vi "PH_Beamline.set Switch State in GUI.vi"(0 "i ref in":refnum<vi>, 1 "Boolean GUI Ref":refnum<vi>, 2 "Picture GUI Ref":refnum<vi>, 3 "Status":T1 items=["no info", "off/false/out", "on/true/in", "Failure", "Alarm", "Status 1", "Status 2", "Status 3"], 4 "no Link?":bool, 5 "error in (no error)":errorcluster) -> (14 "i ref out":refnum<vi>, 19 "error out":errorcluster)   [LabVIEW 2014, in "PH_Beamline.lvlib"]
doc: "This VI writes the incoming information about switches to the GUI."
uses:
  PH_Beamline.lvlib
  PH_StatusHandler/PH_StatusHandler.Status.ctl
  PH_BL-Master/PH_BL-Master.Shutter State.ctl
  PH_Beamline.Switch Instances.ctl
  PH_Common/Picture/PH_Picture.Alignment.ctl
  PH_Common/PH_Common.lvlib
  PH_StatusHandler/PH_StatusHandler.lvlib
  PH_Switch/PH_Switch.lvlib
  PH_Beamline_Common/PH_Beamline_Common.lvlib
  PH_BL-Master/PH_BL-Master.lvlib
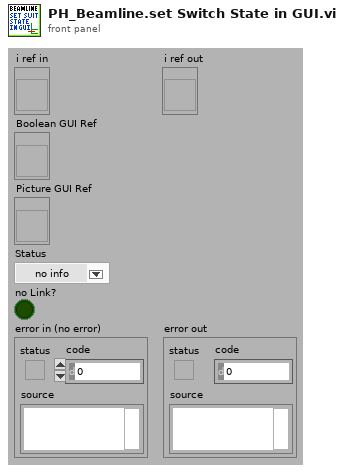
[diagram p1: front panel]
types:
  T1 = typedef "PH_StatusHandler.lvlib/PH_StatusHandler.Status.ctl" = i16
  T2 = typedef "PH_BL-Master.lvlib/PH_BL-Master.Shutter State.ctl" = enum16{"No Link", "No Info", "In", "Out", "in between"}
  T3 = typedef "PH_Beamline.lvlib/PH_Beamline.Switch Instances.ctl" = string
  T4 = typedef "PH_Common.lvlib/PH_Picture.Alignment.ctl" = enum16{"neutral", "left", "right", "up", "down", "vertical", "horizontal", "left down to right up", "left up to right down"}
  T5 = typedef "PH_Beamline.lvlib/PH_Beamline.i attribute.ctl" = cluster{"GUI Refs":cluster{"PA ok":refnum<vi>, "MA ok":refnum<vi>, "fs FE ok":refnum<vi>, "ns FE ok":refnum<vi>, "PA ED ok":refnum<vi>, "MAS ok":refnum<vi>, "Booster ok":refnum<vi>, "Mirrortower ok":refnum<vi>, "In.-Box ok":refnum<vi>, "Compressor ok":refnum<vi>, "Experiment LB ok":refnum<vi>, "Experiment LL ok":refnum<vi>, "PHELIX_Beckhoff_Watchdog":refnum<vi>, "Shutters closed":refnum<vi>, "uOPA ok":refnum<vi>, "Vacuum no shotcond Comp LB":refnum<vi>}, "Refs BL MA":refnum<vi>[], "Refs BL MA-IB":refnum<vi>[], "Refs BL fs":refnum<vi>[], "Refs BL PA ED":refnum<vi>[], "Refs BL MAS":refnum<vi>[], "Refs BL Boo":refnum<vi>[], "Refs BL ns":refnum<vi>[], "Refs BL Mirrortower":refnum<vi>[], "Refs BL Compressor":refnum<vi>[], "Refs BL Exp LB":refnum<vi>[], "Radiation Safety":cluster{"Exp Laserbay":cluster{"Ref Op Mode":refnum<vi>, "Ref Laserbay evacuated":refnum<vi>, "Tagname LB evacuated":string, "Shot Mode":T6, "Laserbay evacuated?":i32, "Tagname HV room locked":string, "HV room locked?":i32, "Ref HV room locked":refnum<vi>, "Tagname bridged?":string, "Ref Bridge":refnum<vi>, "I<1E18W/cm²":bool}, "Exp Laserlab":cluster{"Ref Op Mode":refnum<vi>, "Ref Laserlab evacuated":refnum<vi>, "Tagname LL evacuated":string, "Shot Mode":T6, "Laserlab evacuated?":i32, "Tagname bridged?":string, "Ref Bridge":refnum<vi>, "I<1E18W/cm²":bool}}, "Refs BL LL":refnum<vi>[], "PP Igni Heating GUI Refs":refnum<vi>[], "PP Igni Heating Tagnames ":string[], "Refs BL PA":cluster{"undelayed Line before Shutter":refnum<vi>[], "undelayed Line after Shutter":refnum<vi>[], "before Bypass":refnum<vi>[], "delayed Line before Shutter":refnum<vi>[], "delayed Line after Shutter":refnum<vi>[], "before Shutter Input":refnum<vi>[], "after Shutter Input":refnum<vi>[], "Bypass":refnum<vi>[], "before Shutter Exit":refnum<vi>[], "after Shutter Exit":refnum<vi>[], "to MA":refnum<vi>[], "to Lab":refnum<vi>[]}, "BL":cluster{"YLF_BL_Status":i32, "fs_BL_Status":i32, "fs_YLF_BL_Status":i32, "ns_BL_Status":i32, "PA_Input_BL_Status":i32, "PA_UnDelay_BL_Status":i32, "PA_Delay_BL_Status":i32, "PA_BL_Status":i32, "PA_Bypass_BL_Status":i32, "PA_Exit_BL_Status":i32, "PA_LL_BL_Status":i32, "LL_BL_Status":i32, "PA_MA_BL_Status":i32, "MA_Exit_BL_Status":i32, "MA_Z6_BL_Status":i32, "Z6_BL_Status":i32, "MA_LB_BL_Status":i32, "LB_TB2_BL_Status":i32, "PA_before_Bypass_BL_Status":i32, "LB_TB3_BL_Status":i32}, "State Subsystems":cluster{"PA":bool, "MA":bool, "ns FE":bool, "fs FE":bool, "PA ED":bool, "In.-Box":bool, "MAS":bool, "Booster":bool, "Mirrortower":bool, "Compressor":bool, "Experiment LB":bool, "Experiment LL":bool, "uOPA":bool}, "Status Subscriber Information":T7, "Refs BL uOPA":refnum<vi>[], "PA_Input_2_Beam_6PWpGUI not linked?":bool, "PA_Input_Delay_6PGUI not linked?":bool, "Settings":T10}
  T6 = typedef "PH_Beamline.lvlib/PH_Beamline.Operation Mode.ctl" = i32
  T7 = typedef "PH_Beamline.lvlib/PH_Beamline.Status Subscriber Information.ctl" = cluster{"fs Swich YLF":T8, "fs Exit Shutter":T8, "ns Exit Shutter":T8, "PA Input Shutter":T8, "PA PC WP":T8, "PA PC WP 2":T8, "PA Bypass In":T8, "PA Bypass Out":T8, "PA CH 1":T8, "PA delayed":T8, "PA non delayed":T8, "PA Exit Shutter":T8, "PA Switch Lab":T8, "PA Bridge CH Input MA":T8, "MA Diffusor IB":T8, "MA IB Ready":T8, "MA CH 1":T8, "MA CH 2":T8, "MA CH 3":T8, "MA CH 4":T8, "MA Shutter Align Cam":T8, "MA Position MM5":T8, "Calorimeter Switch":T8, "BL Z6 CH 9":T8, "BL Z6 Beamdump":T8, "BL Z6 Shutter":T8, "COS Sensitivity Switch":T8, "Exp LB Shutter":T8, "Exp LB TB 2":T8, "Exp LB TB 3":T8, "PA LL Input CH":T8, "PA LL Output CH":T8, "LL Comp Input Shutter":T8, "LL Comp Output Shutter":T8, "LL Comp FF Shutter":T8, "Exp LL Shutter":T8, "MA IM In IB":T8, "MA IM Out IB":T8, "MA DB In IB":T8, "MA DB Out IB":T8, "Exp LB Shutter Interlock":T8, "Exp LL Shutter Interlock":T8, "MM1 Force Sensor":T8}
  T8 = typedef "PH_BL-Master.lvlib/PH_BL-Master.Status Subscriber Information.ctl" = cluster{"Index of element":i32, "Attributeset":T9}
  T9 = typedef "PH_BL-Master.lvlib/PH_BL-Master.Attribute Set.ctl" = enum16{"Boolean Status Service Subscriber", "Picture Status Service Subscriber"}
  T10 = typedef "PH_Beamline_Chief.lvlib/PH_Beamline_Chief.Settings.ctl" = cluster{"PA Doublepass Mode":bool, "Compressor Vaccuum LB not relevant":bool, "Windowshutter TB2 not relevant":bool, "Windowshutter TB3 not relevant":bool}
  T11 = typedef "PH_BL-Master.lvlib/PH_BL-Master.i attribute.ctl" = cluster{"Remote controlled":bool, "Boolean Condition Service Subscriber":refnum<vi>[], "Picture Condition Service Subscriber":refnum<vi>[], "R2S":cluster{"GUI Ref":refnum<vi>, "State":bool}, "Vacua":cluster{"GUI Ref":refnum<vi>, "Limit":dbl, "Curr Value":dbl, "in range":bool}[], "O2 Inspection":cluster{"GUI Ref":refnum<vi>, "Concentration":dbl, "State":T1}[], "Boolean Status Service Subscriber":cluster{"GUI Ref":refnum<vi>, "Status":T1, "no Link?":bool, "Status Subscriber Class":T12}[], "Picture Status Service Subscriber":cluster{"GUI Ref":refnum<vi>, "Status":T1, "no Link?":bool, "Status Subscriber Class":T12}[], "6P 4Q Service Subscriber":cluster{"GUI Ref":refnum<vi>, "Selector":T13, "no Link?":bool}[], "Index of latest 6P 4Q changing Instance":i32, "Index of latest Picture Status changing Instance":i32, "Index of latest Boolean Status changing Instance":i32, "Vision ID on same Node":string, "Start Phase over?":bool, "GUI Ref Delete":refnum<vi>}
  T12 = typedef "PH_BL-Master.lvlib/PH_BL-Master.Status Subscriber Class.ctl" = enum16{"unknown", "Switch", "BB", "6P Switch", "Switch GUI", "Switch and 6P State", "Force Sensor"}
  T13 = typedef "PH_4_Pos_Selector.lvlib/PH_4_Pos_Selector.Position Selector.ctl" = u16
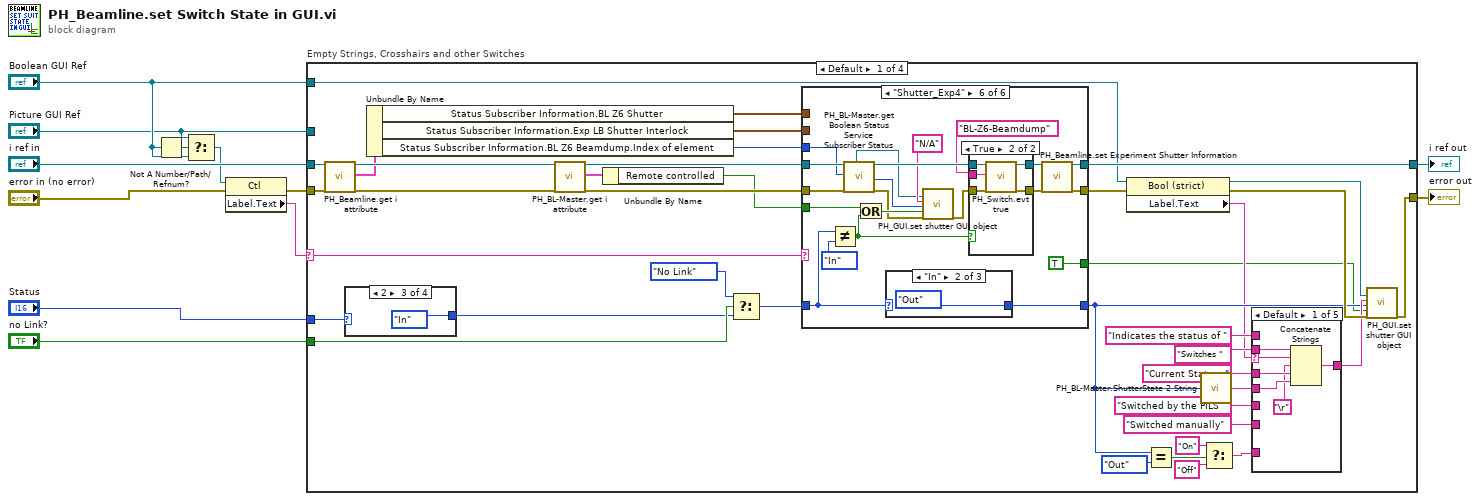
[diagram p0: block diagram]
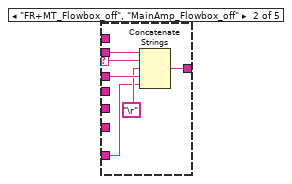
[diagram p2: hidden frame]
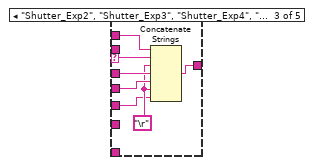
[diagram p3: hidden frame]
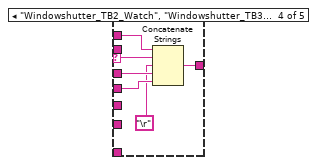
[diagram p4: hidden frame]
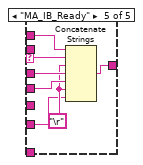
[diagram p5: hidden frame]
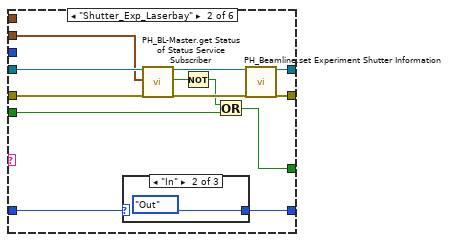
[diagram p7: hidden frame]
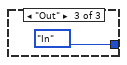
[diagram p9: hidden frame]
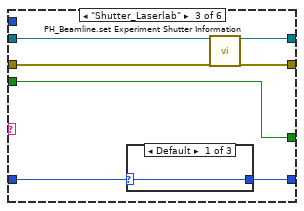
[diagram p10: hidden frame]
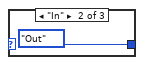
[diagram p11: hidden frame]
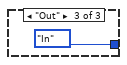
[diagram p12: hidden frame]
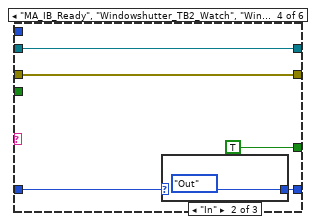
[diagram p13: hidden frame]
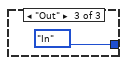
[diagram p15: hidden frame]
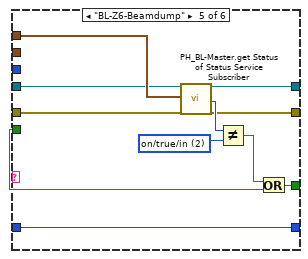
[diagram p16: hidden frame]
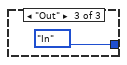
[diagram p18: hidden frame]
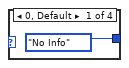
[diagram p20: hidden frame]
diagram:
  n1 = Not A Number/Path/Refnum?(number/path/refnum="Boolean GUI Ref") -> (NaN/Path/Refnum?=w4:bool)
  n2 = Select(t="Picture GUI Ref", s=w4, f="Boolean GUI Ref") -> (s? t:f=w3:refnum<vi>)
  n3 = property class="Ctl"(reference=w3, error in="error in (no error)") -> (error out=w1:errorcluster, "Label.Text"=w2:string)  [unwired: 1 out]
  n4 = case "Empty Strings, Crosshairs and other Switches" shown="Default" w2 {
    selector: w2 -> [w43 _ w178 w192]
    tunnel: w1 -> [w51 w168 w174 w185]
    tunnel: "i ref in" -> [w19 w172 w181 w193]
    tunnel: "Status" -> [w50 w171 w180 w190]
    tunnel: "no Link?" -> [w49 w170 _ _]
    tunnel: [w48 w173 w182 w194] -> w11
    tunnel: [w47 w172 w181 w193] -> w10
    tunnel: "Boolean GUI Ref" -> [w25 _ _ _]
    tunnel: "Picture GUI Ref" -> [_ w169 w175 w186]
    frame Default {
      n5 = call "PH_Beamline.get i attribute.vi"("i ref in"=w19, "error in (no error)"=w51) -> ("i ref out"=w18:refnum<vi>, "i attribute"=w17:T5, "error out"=w20:errorcluster)  [unwired: 15 in]
      n6 = case shown="2" w50 {
        tunnel: [PH_BL-Master.Shutter_State."No Info" ("Shutter State") PH_BL-Master.Shutter_State."Out" ("Shutter State") PH_BL-Master.Shutter_State."In" ("Shutter State") PH_BL-Master.Shutter_State."in between" ("Shutter State")] -> w45
        frame 0, Default {
        }
        frame 1 {
        }
        frame 2 {
        }
        frame 5 {
        }
      }
      n7 = Unbundle By Name(w17) -> ("Status Subscriber Information.BL Z6 Shutter"=w14:T8, "Status Subscriber Information.Exp LB Shutter Interlock"=w15:T8, "Status Subscriber Information.BL Z6 Beamdump.Index of element"=w16:i32)
      n8 = call "PH_BL-Master.get i attribute.vi"("i ref in"=w18, "error in (no error)"=w20) -> ("i ref out"=w26:refnum<vi>, "i attribute"=w22:T11, "error out"=w27:errorcluster)  [unwired: 15 in]
      n9 = Unbundle By Name(w22) -> ("Remote controlled"=w13:bool)
      n10 = Select(t=PH_BL-Master.Shutter_State."No Link" ("Shutter State"), s=w49, f=w45) -> (s? t:f=w44:T2)
      n11 = case shown="\"Shutter_Exp4\"" w43 {
        tunnel: w13 -> [w87 w97 w110 _ w125 w151]
        tunnel: [w87 w96 w110 TRUE w132 TRUE] -> w21
        tunnel: w26 -> [w86 w90 w109 w118 w123 w148]
        tunnel: [w86 w91 w106 w118 w130 w135] -> w47
        tunnel: w27 -> [w85 w89 w105 w117 w122 w149]
        tunnel: [w85 w93 w104 w117 w129 w137] -> w23
        tunnel: w44 -> [w84 w95 w108 w115 w128 w143]
        tunnel: [w84 w94 w107 w114 w128 w142] -> w34
        tunnel: w16 -> [_ _ _ _ _ w133]
        tunnel: w15 -> [_ w88 _ _ _ _]
        tunnel: w14 -> [_ _ _ _ w124 _]
        frame Default {
        }
        frame "Shutter_Exp_Laserbay" {
          n12 = case shown="\"In\"" w95 {
            selector: w95 -> [w101 _ _]
            tunnel: [w101 PH_BL-Master.Shutter_State."Out" ("Shutter State") PH_BL-Master.Shutter_State."In" ("Shutter State")] -> w94
            frame Default {
            }
            frame "In" {
            }
            frame "Out" {
            }
          }
          n13 = call "PH_BL-Master.get Status of Status Service Subscriber.vi"("i ref in"=w90, "Wanted Status Subscriber Information"=w88, "error in (no error)"=w89) -> ("i ref out"=w92:refnum<vi>, "on/true/in?"=w99:bool, "error out"=w100:errorcluster)  [unwired: 11 in, 3 out]
          n14 = Not(x=w99) -> (.not. x?=w98:bool)
          n15 = Or(x=w98, y=w97) -> (x .or. y?=w96:bool)
          n16 = call "PH_Beamline.set Experiment Shutter Information.vi"("i ref in"=w92, "error in"=w100) -> ("i ref out"=w91:refnum<vi>, "error out"=w93:errorcluster)  [unwired: 16 in]
        }
        frame "Shutter_Laserlab" {
          n17 = case shown="Default" w108 {
            selector: w108 -> [w111 _ _]
            tunnel: [w111 PH_BL-Master.Shutter_State."Out" ("Shutter State") PH_BL-Master.Shutter_State."In" ("Shutter State")] -> w107
            frame Default {
            }
            frame "In" {
            }
            frame "Out" {
            }
          }
          n18 = call "PH_Beamline.set Experiment Shutter Information.vi"("i ref in"=w109, "error in"=w105) -> ("i ref out"=w106:refnum<vi>, "error out"=w104:errorcluster)  [unwired: 16 in]
        }
        frame "MA_IB_Ready", "Windowshutter_TB2_Watch", "Windowshutter_TB3_Watch" {
          n19 = case shown="\"In\"" w115 {
            selector: w115 -> [w119 _ _]
            tunnel: [w119 PH_BL-Master.Shutter_State."Out" ("Shutter State") PH_BL-Master.Shutter_State."In" ("Shutter State")] -> w114
            frame Default {
            }
            frame "In" {
            }
            frame "Out" {
            }
          }
        }
        frame "BL-Z6-Beamdump" {
          w127 = T1 2 items=["no info", "off/false/out", "on/true/in", "Failure", "Alarm", "Status 1", "Status 2", "Status 3"] ("Subscriber State")
          n20 = call "PH_BL-Master.get Status of Status Service Subscriber.vi"("i ref in"=w123, "Wanted Status Subscriber Information"=w124, "error in (no error)"=w122) -> ("i ref out"=w130:refnum<vi>, "Status"=w131:T1, "error out"=w129:errorcluster)  [unwired: 11 in, 3 out]
          n21 = Not Equal?(x=w131, y=w127) -> (x != y?=w126:bool)
          n22 = Or(x=w126, y=w125) -> (x .or. y?=w132:bool)
        }
        frame "Shutter_Exp4" {
          n23 = Not Equal?(x=w143, y=PH_BL-Master.Shutter_State."In" ("State")) -> (x != y?=w141:bool)
          n24 = call "PH_BL-Master.get Boolean Status Service Subscriber Status.vi"("i ref in"=w148, "Index of wanted element"=w133, "error in (no error)"=w149) -> ("Wanted Boolean Ref"=w139:refnum<vi>, "i ref out"=w145:refnum<vi>, "Subscriber State"=w147:T1, "error out"=w138:errorcluster)  [unwired: 8 in, 5 out]
          n25 = Or(x=w151, y=w141) -> (x .or. y?=w150:bool)
          n26 = case shown="\"In\"" w143 {
            selector: w143 -> [w154 _ _]
            tunnel: [w154 PH_BL-Master.Shutter_State."Out" ("Shutter State") PH_BL-Master.Shutter_State."In" ("Shutter State")] -> w142
            frame Default {
            }
            frame "In" {
            }
            frame "Out" {
            }
          }
          n27 = call "PH_GUI.set shutter GUI object.vi"("Wanted Boolean Ref"=w139, "Tip Strip"="N/A", "Shutter State"=w147, "Disabled? (false)"=w150, "error in (no error)"=w138) -> ("error out"=w144:errorcluster)  [unwired: 14 in]
          n28 = case shown="True" w141 {
            tunnel: [w157 w163] -> w146
            tunnel: [w158 w162] -> w136
            tunnel: w145 -> [w158 w161]
            tunnel: w144 -> [w157 w160]
            tunnel: T3 "BL-Z6-Beamdump" ("Switch Instance") -> [_ w159]
            frame False {
            }
            frame True {
              n29 = call "PH_Switch.evt true.vi"("i ref in"=w161, "Instance"=w159, "error in (no error)"=w160) -> ("i ref out"=w162:refnum<vi>, "error out"=w163:errorcluster)  [unwired: 15 in]
            }
          }
          n30 = call "PH_Beamline.set Experiment Shutter Information.vi"("i ref in"=w136, "error in"=w146) -> ("i ref out"=w135:refnum<vi>, "error out"=w137:errorcluster)  [unwired: 16 in]
        }
      }
      n31 = property class="Bool (strict)"(reference=w25, error in=w23) -> (reference out=w37:refnum<vi>, error out=w36:errorcluster, "Label.Text"=w24:string)
      n32 = Equal?(x=w34, y=PH_BL-Master.Shutter_State."Out") -> (x = y?=w31:bool)
      n33 = call "PH_BL-Master.ShutterState 2 String.vi"("Shutter State"=w34) -> ("String"=w38:string)
      n34 = Select(t="On", s=w31, f="Off") -> (s? t:f=w28:string)
      n35 = case shown="Default" w24 {
        selector: w24 -> [w52 w59 w67 w73 w80]
        tunnel: [w57 w63 w70 w76 w83] -> w35
        tunnel: "Current Status: " ("string") -> [w56 w62 w69 w75 w82]
        tunnel: w38 -> [w55 _ w68 w74 w81]
        tunnel: "Switches " ("string") -> [w53 w60 _ _ _]
        tunnel: "Indicates the status of " ("string") -> [_ _ w66 w72 w79]
        tunnel: "Switched by the PILS" ("string") -> [_ _ w64 _ _]
        tunnel: "Switched manually" ("string") -> [_ _ _ _ w77]
        tunnel: w28 -> [_ w58 _ _ _]
        frame Default {
          n36 = Concatenate Strings(w53, w52, "\r", w56, w55) -> (w57:string)
        }
        frame "FR+MT_Flowbox_off", "MainAmp_Flowbox_off" {
          n37 = Concatenate Strings(w60, w59, "\r", w62, w58) -> (w63:string)
        }
        frame "Shutter_Exp2", "Shutter_Exp3", "Shutter_Exp4", "Sutter_Exp1" {
          w65 = "\r"
          n38 = Concatenate Strings(w66, w67, w65, w69, w68, w65, w64) -> (w70:string)
        }
        frame "Windowshutter_TB2_Watch", "Windowshutter_TB3_Watch" {
          n39 = Concatenate Strings(w72, w73, "\r", w75, w74) -> (w76:string)
        }
        frame "MA_IB_Ready" {
          w78 = "\r"
          n40 = Concatenate Strings(w79, w80, w78, w82, w81, w78, w77) -> (w83:string)
        }
      }
      n41 = call "PH_GUI.set shutter GUI object.vi"("Wanted Boolean Ref"=w37, "Tip Strip"=w35, "Shutter State"=w34, "Disabled? (false)"=w21, "error in (no error)"=w36) -> ("error out"=w48:errorcluster)  [unwired: 14 in]
    }
    frame "BL-Z6-CH9", "MA01_CH1", "MA01_CH2", "MA01_CH3", "MA01_CH4" {
      n42 = call "PH_Beamline_Common.set Crosshair.vi"("CtlRef"=w169, "State"=w171, "no link"=w170, "error in (no error)"=w168) -> ("error out"=w173:errorcluster)  [unwired: 15 in]
    }
    frame "MA_InB_IM_In_Switch", "MA_InB_IM_Out_Switch" {
      n43 = case shown="\"MA_InB_IM_In_Switch\"" w178 {
        tunnel: [PH_Picture.Alignment."left down to right up" ("Alignment (left down to right up)") PH_Picture.Alignment."left up to right down" ("Alignment (left down to right up)")] -> w177
        frame Default {
        }
        frame "MA_InB_IM_In_Switch" {
        }
      }
      n44 = call "PH_Beamline_Common.set Mirror.vi"("Alignment (left down to right up)"=w177, "CtlRef"=w175, "Status (on/true/in)"=w180, "GUI Instance does not exist or here?"=TRUE, "error in (no error)"=w174, "Tip Strip (N/A)"="Switches") -> ("error out"=w182:errorcluster)  [unwired: 13 in]
    }
    frame "PA_Bypass_In", "PA_Bypass_Out" {
      w189 = T1 1 items=["no info", "off/false/out", "on/true/in", "Failure", "Alarm", "Status 1", "Status 2", "Status 3"] ("y")
      n45 = case shown="\"PA_Bypass_Out\"" w192 {
        tunnel: [PH_Picture.Alignment."left down to right up" ("Alignment (left down to right up)") PH_Picture.Alignment."left up to right down" ("Alignment (left down to right up)")] -> w191
        frame Default {
        }
        frame "PA_Bypass_Out" {
        }
      }
      n46 = Equal?(x=w190, y=w189) -> (x = y?=w188:bool)
      n47 = call "PH_Beamline_Common.set Mirror.vi"("Alignment (left down to right up)"=w191, "CtlRef"=w186, "Status (on/true/in)"=w190, "GUI Instance does not exist or here?"=w188, "error in (no error)"=w185, "Tip Strip (N/A)"="Indicates the status of") -> ("error out"=w194:errorcluster)  [unwired: 13 in]
    }
  }
  "error out" <- w11
  "i ref out" <- w10
